vi "AddGlyphtoGManager.vi"(8 "error in":errorcluster, 10 "glyph manager":T1, 11 "Abstract Engine in":refnum<class "Abstract Engine.lvclass">) -> (0 "error out":errorcluster, 2 "glyph manager out":T1, 3 "Abstract Engine out":refnum<class "Abstract Engine.lvclass">)   [LabVIEW 2025, in "Abstract Engine.lvlib" / "Abstract Engine.lvclass"]
doc: "Copyright 2017 National Instruments Corporation\n\nLicensed under the Apache License, Version 2.0 (the \"License\"); you may not use this file except in compliance with the License. You may obtain a copy of the License at http://www.apache.org/licenses/LICENSE-2.0\nUnless required by applicable law or agreed to in writing, software distributed under the License is distributed on an \"AS IS\" BASIS, WITHOUT WARRANTIES OR CONDITIONS OF ANY KIND, either express or implied. See the License for the specific language governing permissions and limitations under the License."
uses:
  Abstract Engine.lvclass
  Users/Public/Documents/Sandia National Labs/TSS Plugin/CEF.lvlibp/serializable node/CEF_serializable node.lvclass
  Users/Public/Documents/Sandia National Labs/TSS Plugin/CEF.lvlibp
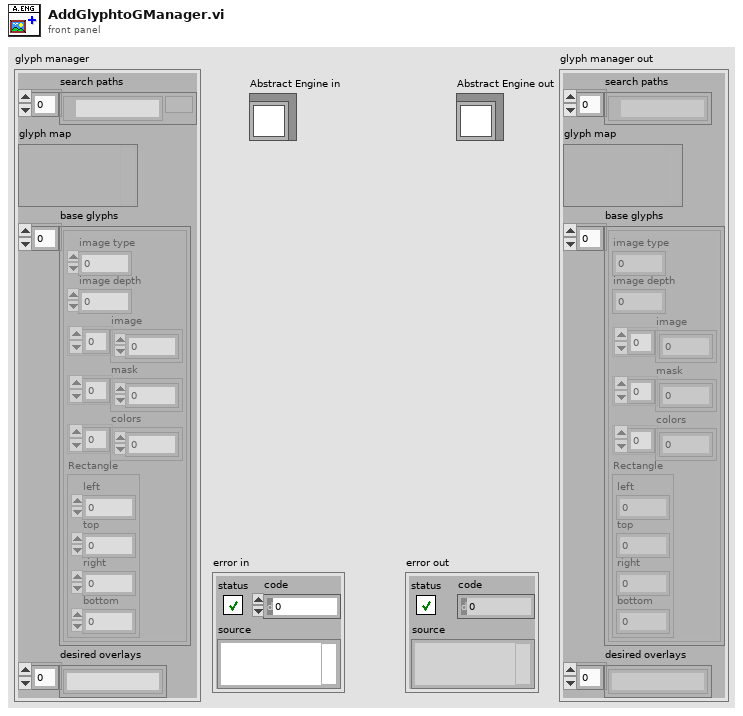
[diagram p1: front panel]
types:
  T1 = cluster{"search paths":path[], "glyph map":variant, "base glyphs":cluster{"image type":i32, "image depth":i32, "image":u8[], "mask":u8[], "colors":u32[], "Rectangle":cluster{"left":i16, "top":i16, "right":i16, "bottom":i16}}[], "desired overlays":string[]}
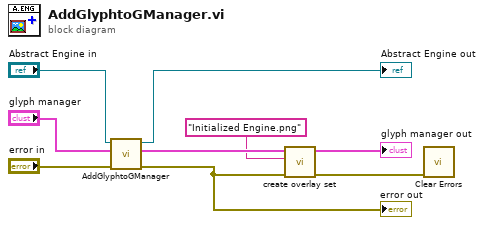
[diagram p0: block diagram]
diagram:
  n1 = call-parent "AddGlyphtoGManager.vi"("error in"="error in", "glyph manager"="glyph manager", "CEF_serializable node in"="Abstract Engine in") -> ("error out"=w2:errorcluster, "glyph manager out"=w5:T1, "CEF_serializable node out"=→"Abstract Engine out":refnum<class "Abstract Engine.lvclass">)  [unwired: 6 in]
  "error out" <- w2
  n2 = call "create overlay set.vi"("error in"=w2, "overlay glyph"="Initialized Engine.png" ("overlay"), "glyph manager in"=w5) -> ("error out"=w1:errorcluster, "glyph manager out"=→"glyph manager out":T1)  [unwired: 7 in]
  n3 = call <vilib>:"Clear Errors.vi"("error in (no error)"=w1) -> ()  [unwired: 5 in, 2 out]
